vi "Color Components Range Extender.vi"(11 "Color Components":T1={"Hue"={110.0, 142.0}, "Sat"={138.0, 255.0}, "Val"={139.0, 198.0}} {"Val" scale=0.0..255.0; "Sat" scale=0.0..255.0; "Hue" scale=0.0..255.0 scale format="%#_3g"}) -> (3 "Color Components 2":T1={"Hue"={110.0, 142.0}, "Sat"={138.0, 255.0}, "Val"={139.0, 198.0}} {"Val" scale=0.0..255.0; "Sat" scale=0.0..255.0; "Hue" scale=0.0..255.0 scale format="%#_3g"})   [LabVIEW 2013]
panel:
  in  "Ranging colors":dbl=50.0 format="%#_13g"
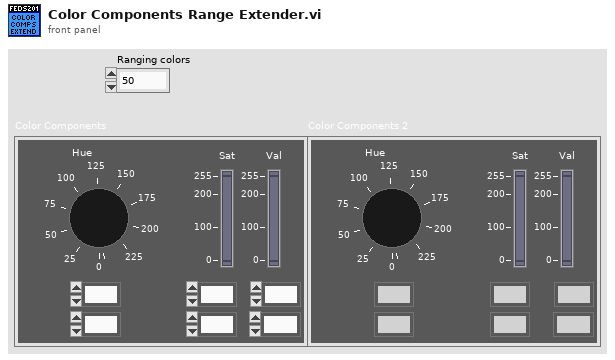
[diagram p1: front panel]
types:
  T1 = cluster{"Hue":cluster{dbl, dbl}, "Sat":cluster{dbl, dbl}, "Val":cluster{dbl, dbl}}
  T2 = cluster{cluster{dbl, "y":dbl}, cluster{dbl, "y":dbl}, cluster{dbl, "y":dbl}}
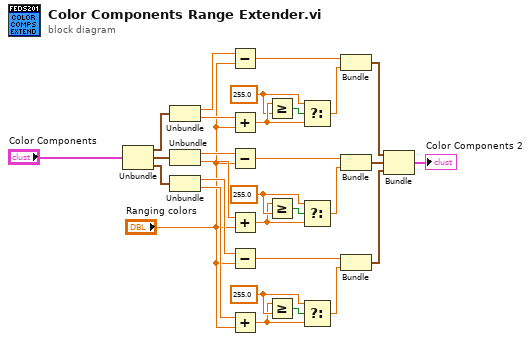
[diagram p0: block diagram]
diagram:
  w11 = 255.0 ("y")
  w16 = 255.0 ("y")
  w17 = 255.0 ("y")
  n1 = Unbundle("Color Components") -> ("Hue"=w4:cluster{dbl, dbl}, "Sat"=w3:cluster{dbl, dbl}, "Val"=w2:cluster{dbl, dbl})
  n2 = Unbundle(w4) -> (w23:dbl, w24:dbl)
  n3 = Unbundle(w3) -> (w26:dbl, w25:dbl)
  n4 = Unbundle(w2) -> (w30:dbl, w29:dbl)
  n5 = Subtract(x=w23, y="Ranging colors") -> (x-y=w22:dbl)
  n6 = Add(x=w24, y="Ranging colors") -> (x+y=w19:dbl)
  n7 = Subtract(x=w26, y="Ranging colors") -> (x-y=w27:dbl)
  n8 = Add(x=w25, y="Ranging colors") -> (x+y=w14:dbl)
  n9 = Subtract(x=w30, y="Ranging colors") -> (x-y=w28:dbl)
  n10 = Add(x=w29, y="Ranging colors") -> (x+y=w10:dbl)
  n11 = Greater Or Equal?(x=w19, y=w17) -> (x >= y?=w20:bool)
  n12 = Greater Or Equal?(x=w14, y=w16) -> (x >= y?=w15:bool)
  n13 = Greater Or Equal?(x=w10, y=w11) -> (x >= y?=w12:bool)
  n14 = Select(t=w17, s=w20, f=w19) -> (s? t:f=w18:dbl)
  n15 = Select(t=w16, s=w15, f=w14) -> (s? t:f=w13:dbl)
  n16 = Select(t=w11, s=w12, f=w10) -> (s? t:f=w9:dbl)
  n17 = Bundle(w22, "y"=w18) -> (w8:cluster{dbl, "y":dbl})  [unwired: 1 in]
  n18 = Bundle(w27, "y"=w13) -> (w7:cluster{dbl, "y":dbl})  [unwired: 1 in]
  n19 = Bundle(w28, "y"=w9) -> (w6:cluster{dbl, "y":dbl})  [unwired: 1 in]
  n20 = Bundle(w8, w7, w6) -> (→"Color Components 2":T2)  [unwired: 1 in]
